vi "Remove NaN.vi"(11 "Value In":sgl) -> (3 "Value Out":sgl)   [LabVIEW 2015, in "ECS-RT.lvlib"]
uses:
  ECS-RT.lvlib
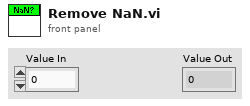
[diagram p1: front panel]
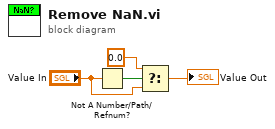
[diagram p0: block diagram]
diagram:
  n1 = Not A Number/Path/Refnum?(number/path/refnum="Value In") -> (NaN/Path/Refnum?=w1:bool)
  n2 = Select(t=sgl 0.0, s=w1, f="Value In") -> (s? t:f=→"Value Out":sgl)
